vi "Save Result Parameters_Temperature.vi"(0 "report In":T2, 1 "SetupFile_Path":string, 2 "Measure Station Setup":T1 {"scopeResistOhm" format="%.2f"; "scopeCapacityF" format="%.2e"}, 3 "Probe Name":string, 4 "Moving OSTL enable":bool, 5 "WCS":bool) -> (7 "next cell bottom-left":cluster{"row":i32, "column":i32}, 8 "report out":T2)   [LabVIEW 2016]
uses:
  <vilib>/Utility/NIReport.llb/Generate Report Object Reference.ctl
  <vilib>/Utility/NIReport.llb/NI_report.lvclass
  <vilib>/addons/_office/excel.llb/Excel Easy Table (str).vi
  TypeDefinitions/StationCmdsGlobal.vi
  <vilib>/addons/_office/NI_ReportGenerationToolkit.lvlib
  <vilib>/Utility/NIReport.llb/Excel/NI_Excel.lvclass
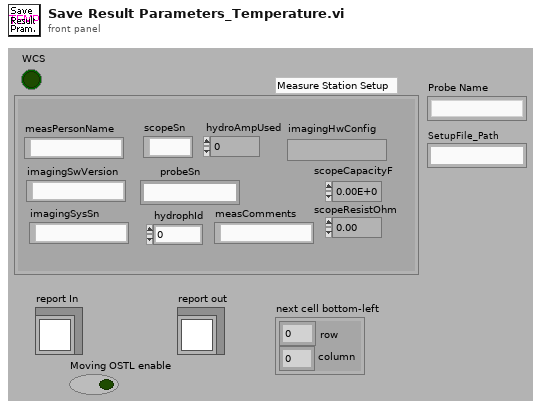
[diagram p1: front panel]
types:
  T1 = cluster{"imagingSwVersion":string, "measPurpose":string, "measComments":string, "probeId":i16, "hydrophId":i16, "probeSn":string, "measPersonName":string, "imagingSysSn":string, "labviewSwVersion":string, "scopeSn":string, "scopeCapacityF":sgl, "scopeResistOhm":sgl, "hydroAmpUsed":i8, "imagingHwConfig":string, "measSSId":i32}
  T2 = typedef "Generate Report Object Reference.ctl" = refnum<class "NI_report.lvclass">
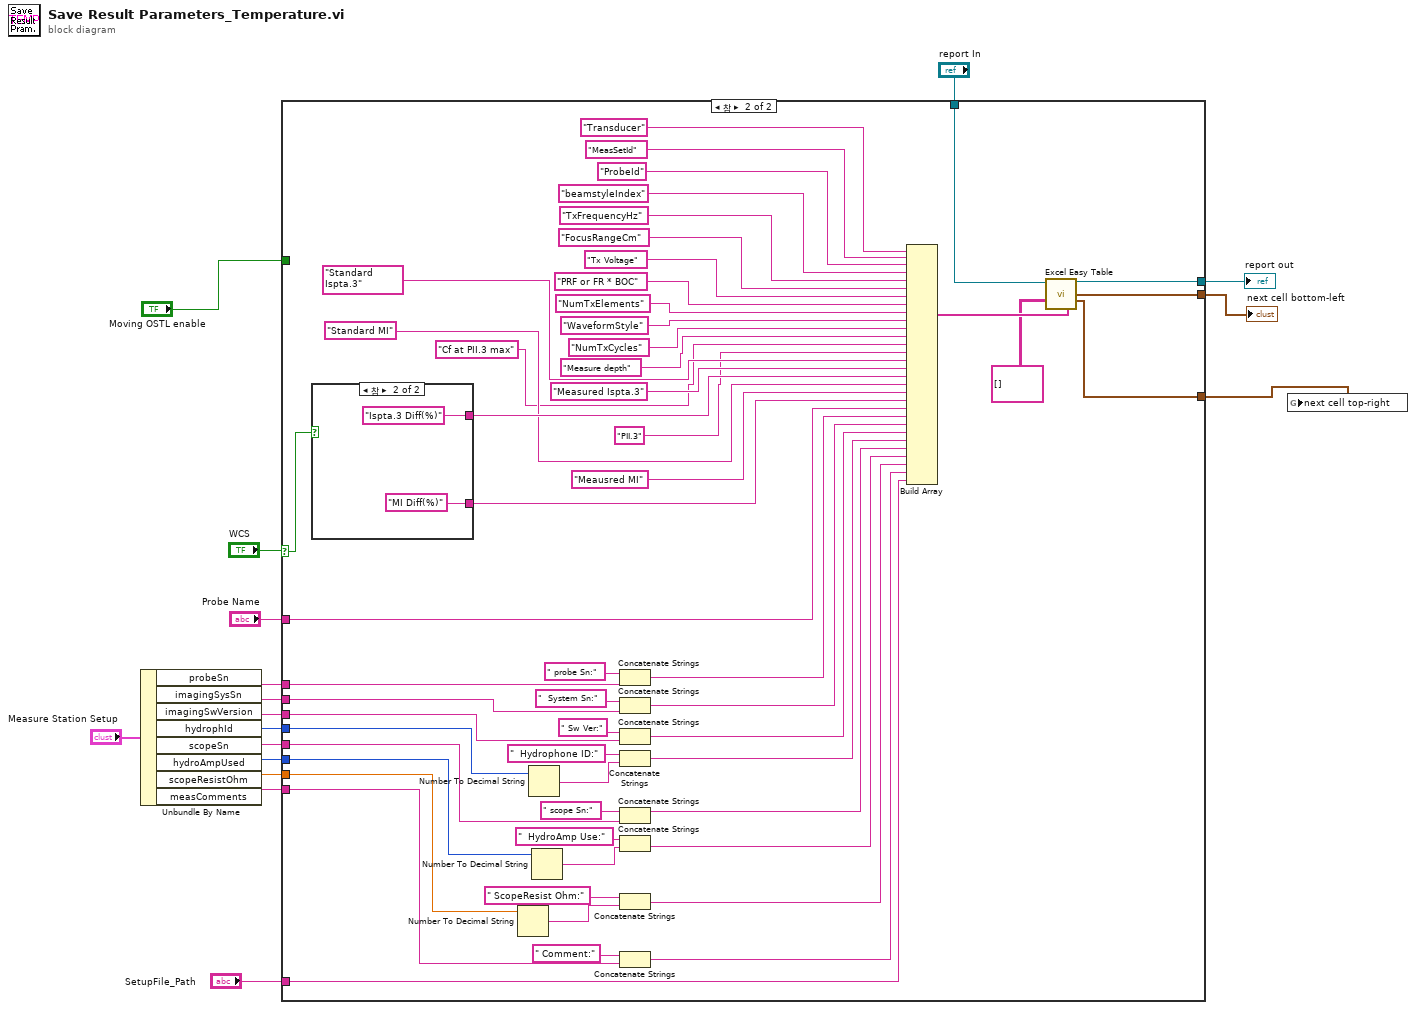
[diagram p0: block diagram]
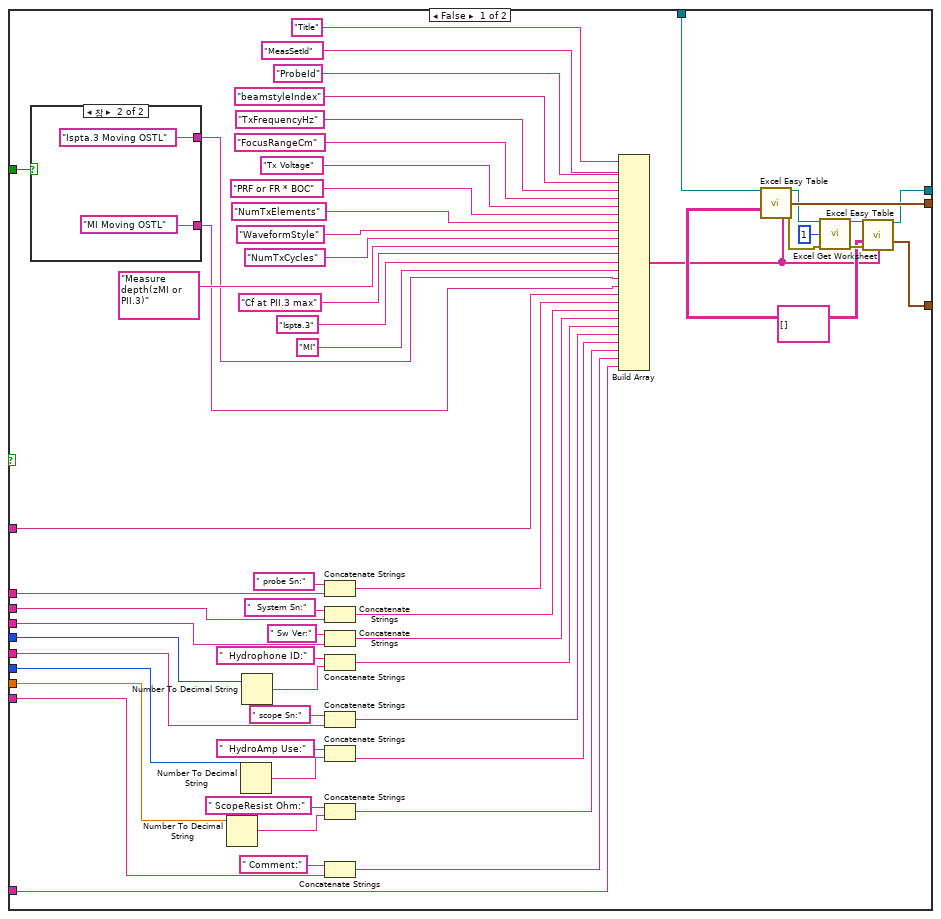
[diagram p2: hidden frame]
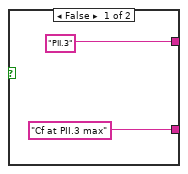
[diagram p3: hidden frame]
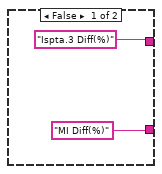
[diagram p4: hidden frame]
diagram:
  n1 = Unbundle By Name("Measure Station Setup") -> ("probeSn"=w13:string, "imagingSysSn"=w12:string, "imagingSwVersion"=w11:string, "hydrophId"=w10:i16, "scopeSn"=w8:string, "hydroAmpUsed"=w7:i8, "scopeResistOhm"=w6:sgl, "measComments"=w5:string)
  n2 = case shown="참" "WCS" {
    selector: "WCS" -> [_ w89]
    tunnel: [w23 w102] -> w16
    tunnel: "report In" -> [w31 w103]
    tunnel: [w33 w99] -> w14
    tunnel: w13 -> [w43 w98]
    tunnel: w12 -> [w42 w97]
    tunnel: w11 -> [w41 w96]
    tunnel: w10 -> [w40 w95]
    tunnel: w8 -> [w39 w94]
    tunnel: w7 -> [w38 w93]
    tunnel: w6 -> [w36 w92]
    tunnel: w5 -> [w37 w91]
    tunnel: "Probe Name" -> [w44 w90]
    tunnel: "SetupFile_Path" -> [w35 w86]
    tunnel: "Moving OSTL enable" -> [w34 _]
    tunnel: [w24 w83] -> w1
    frame False {
      w26 = string[][] [] ("numerical data")
      n3 = case shown="참" w34 {
        tunnel: ["PII.3" ("element") "Ispta.3 Moving OSTL" ("element")] -> w19
        tunnel: ["Cf at PII.3 max" ("element") "MI Moving OSTL" ("element")] -> w18
        frame False {
        }
        frame True {
        }
      }
      n4 = Number To Decimal String(number=w36) -> (decimal integer string=w54:string)  [unwired: 1 in]
      n5 = Number To Decimal String(number=w38) -> (decimal integer string=w56:string)  [unwired: 1 in]
      n6 = Number To Decimal String(number=w40) -> (decimal integer string=w59:string)  [unwired: 1 in]
      n7 = Concatenate Strings(" probe Sn:" ("element"), w43) -> (w52:string)
      n8 = Concatenate Strings("  System Sn:" ("element"), w42) -> (w51:string)
      n9 = Concatenate Strings(" Sw Ver:" ("element"), w41) -> (w50:string)
      n10 = Concatenate Strings("  Hydrophone ID:" ("element"), w59) -> (w49:string)
      n11 = Concatenate Strings(" scope Sn:" ("element"), w39) -> (w48:string)
      n12 = Concatenate Strings("  HydroAmp Use:" ("element"), w56) -> (w47:string)
      n13 = Concatenate Strings(" ScopeResist Ohm:" ("element"), w54) -> (w46:string)
      n14 = Concatenate Strings(" Comment:" ("element"), w37) -> (w45:string)
      n15 = Build Array("Title" ("string"), "MeasSetId" ("string"), "ProbeId" ("string"), "beamstyleIndex" ("string"), "TxFrequencyHz", "FocusRangeCm" ("element"), "Tx Voltage" ("element"), "PRF or FR * BOC" ("element"), "NumTxElements" ("element"), "WaveformStyle" ("element"), "NumTxCycles" ("element"), "Measure depth(zMI or PII.3)" ("element"), "Cf at PII.3 max" ("element"), "Ispta.3" ("element"), "MI" ("element"), w19, w18, w44, w52, w51, w50, w49, w48, w47, w46, w45, w35) -> (w25:string[])
      n16 = call-poly <vilib>:"Excel Easy Table.vi"("report in"=w31, "text data"=w26, "column headers"=w25) -> ("report out"=w30:refnum<class "NI_report.lvclass">, "next cell bottom-left"=w33:cluster{"row":i32, "column":i32}, "error out"=w29:errorcluster)  [unwired: 8 in, 2 out]
      n17 = call <vilib>:"Excel Get Worksheet.vi"("report in"=w30, "worksheet index (0)"=1, "error in (no error)"=w29) -> ("report out"=w28:refnum<class "NI_report.lvclass">, "error out"=w27:errorcluster)  [unwired: 11 in]
      n18 = call-poly <vilib>:"Excel Easy Table.vi"("report in"=w28, "text data"=w26, "error in (no error)"=w27, "row headers"=w25) -> ("report out"=w23:refnum<class "NI_report.lvclass">, "next cell top-right"=w24:cluster{"row":i32, "column":i32})  [unwired: 7 in, 3 out]
    }
    frame True {
      n19 = case shown="참" w89 {
        tunnel: ["Ispta.3 Diff(%)" ("element") "Ispta.3 Diff(%)" ("element")] -> w88
        tunnel: ["MI Diff(%)" ("element") "MI Diff(%)" ("element")] -> w87
        frame False {
        }
        frame True {
        }
      }
      n20 = Number To Decimal String(number=w92) -> (decimal integer string=w113:string)  [unwired: 1 in]
      n21 = Number To Decimal String(number=w95) -> (decimal integer string=w118:string)  [unwired: 1 in]
      n22 = Number To Decimal String(number=w93) -> (decimal integer string=w115:string)  [unwired: 1 in]
      n23 = Concatenate Strings(" probe Sn:" ("element"), w98) -> (w111:string)
      n24 = Concatenate Strings("  System Sn:" ("element"), w97) -> (w110:string)
      n25 = Concatenate Strings(" Sw Ver:" ("element"), w96) -> (w109:string)
      n26 = Concatenate Strings("  Hydrophone ID:" ("element"), w118) -> (w108:string)
      n27 = Concatenate Strings(" scope Sn:" ("element"), w94) -> (w107:string)
      n28 = Concatenate Strings("  HydroAmp Use:" ("element"), w115) -> (w106:string)
      n29 = Concatenate Strings(" ScopeResist Ohm:" ("element"), w113) -> (w105:string)
      n30 = Concatenate Strings(" Comment:" ("element"), w91) -> (w104:string)
      n31 = Build Array("Transducer" ("string"), "MeasSetId" ("string"), "ProbeId" ("string"), "beamstyleIndex" ("string"), "TxFrequencyHz", "FocusRangeCm" ("element"), "Tx Voltage" ("element"), "PRF or FR * BOC" ("element"), "NumTxElements" ("element"), "WaveformStyle" ("element"), "NumTxCycles" ("element"), "Measure depth" ("element"), "Cf at PII.3 max" ("element"), "PII.3" ("element"), "Standard Ispta.3" ("element"), "Measured Ispta.3" ("element"), w88, "Standard MI" ("element"), "Meausred MI" ("element"), w87, w90, w111, w110, w109, w108, w107, w106, w105, w104, w86) -> (w101:string[])
      n32 = call-poly <vilib>:"Excel Easy Table.vi"("report in"=w103, "text data"=string[][] [] ("numerical data"), "column headers"=w101) -> ("report out"=w102:refnum<class "NI_report.lvclass">, "next cell bottom-left"=w99:cluster{"row":i32, "column":i32}, "next cell top-right"=w83:cluster{"row":i32, "column":i32})  [unwired: 8 in, 2 out]
    }
  }
  "report out" <- w16
  "next cell bottom-left" <- w14
  n33 = global write "StationCmdsGlobal.vi" "next cell top-right"(w1) -> ()
